vi "FPGAcode4_NoInit.vi"() -> ()   [LabVIEW 2015]
uses:
  Limits_In.ctl
  Detector_Cluster.ctl
  <vilib>/Platform/TimedLoop/XDataNode/timing_clust.ctl
  <vilib>/Platform/TimedLoop/XDataNode/nitl_modes.ctl
  <vilib>/Platform/TimedLoop/XDataNode/wakeup.ctl
  Correlations.ctl
  <vilib>/rvi/Emulation/niFpgaSctlEmulationGetInTimedLoop.vi
  <vilib>/rvi/Emulation/niFpgaEmulationReportErrorSimple.vi
  <vilib>/rvi/Emulation/niFpgaGetClockAttributes.vi
  <vilib>/rvi/Emulation/niFpgaCriticalErrorInLSC.vi
  <vilib>/rvi/eio/common/nirviEmuTemplateMethod_errors.vi
  <vilib>/rvi/Emulation/niFpgaEmulationIsFPGAContextNoSignature.vi
  <vilib>/rvi/DataTransferAndStorage/Container/Common/niFpgaContainerGetUniqueNameForEmu.vi
  <vilib>/rvi/eio/common/nirviEmuReportErrorAndStop.vi
  <vilib>/rvi/Emulation/niFpgaProcessEmulError.vi
  <vilib>/Platform/TimedLoop/XDataNode/XDataNode.xnode
  <vilib>/eio/EIONode/EIONode.xnode
  <vilib>/rvi/DataTransferAndStorage/Container/XNode/niFpgaContainer.xnode
  <vilib>/rvi/DataTransferAndStorage/Handshake/Emulation/niFpgaHandshakeEmulation.vi
  <vilib>/Platform/TimedLoop/XDataNode/XDNodeRunTimeDep.lvlib
panel:
  in  "User Trigger?":bool
  in  "User Trigger Distance":fxp<+/-,34,18> format="%.3g"
  in  "Charge Error Factor":fxp<+,32,0>=0.19999999995343387 format="%_2g"
  in  "Threshold Factor":fxp<+/-,32,16>=1.149993896484375 format="%.2g"
  in  "Limits":T1={"High Charge Limit"=4.54747350780585e-13, "Low Charge Limit"=0.0, "High Velocity Limit"=262143.0, "Low Velocity Limit"=0.0, "High Mass Limit"=7.27595761248936e-12, "Low Mass Limit"=0.0, "High Voltage"=2200000.0}
  in  "Calibrate":bool=TRUE
  in  "Armed":bool
  in  "One Shot":bool
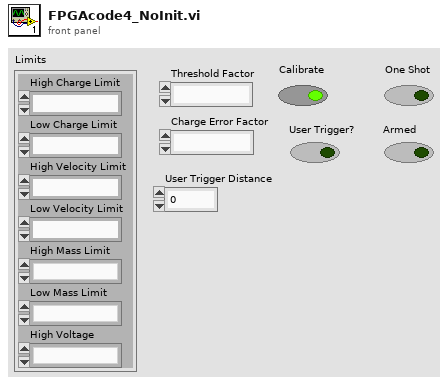
[diagram p1: front panel]
types:
  T1 = typedef "Limits_In.ctl" = cluster{"High Charge Limit":fxp<+,32,-41>, "Low Charge Limit":fxp<+,32,-41>, "High Velocity Limit":fxp<+,18,18>, "Low Velocity Limit":fxp<+,18,18>, "High Mass Limit":fxp<+,32,-37>, "Low Mass Limit":fxp<+,32,-37>, "High Voltage":fxp<+,32,22>}
  T2 = cluster{"[0]":fxp<+,16,1>, "[1]":fxp<+,16,1>, "[2]":fxp<+,16,1>, "[3]":fxp<+,16,1>, "[4]":fxp<+,16,1>, "[5]":fxp<+,16,1>, "[6]":fxp<+,16,1>, "[7]":fxp<+,16,1>, "[8]":fxp<+,16,1>, "[9]":fxp<+,16,1>, "[10]":fxp<+,16,1>}
  T3 = cluster{"[0]":i32, "[1]":i32, "[2]":i32, "[3]":i32, "[4]":i32, "[5]":i32, "[6]":i32, "[7]":i32, "[8]":i32, "[9]":i32, "[10]":i32}
  T4 = cluster{"[0]":cluster{"Detector Max Speed Count":i32, "Detector Min Speed Count":i32, "Gap Max Speed Count":i32, "Gap Min Speed Count":i32}, "[1]":cluster{"Detector Max Speed Count":i32, "Detector Min Speed Count":i32, "Gap Max Speed Count":i32, "Gap Min Speed Count":i32}, "[2]":cluster{"Detector Max Speed Count":i32, "Detector Min Speed Count":i32, "Gap Max Speed Count":i32, "Gap Min Speed Count":i32}, "[3]":cluster{"Detector Max Speed Count":i32, "Detector Min Speed Count":i32, "Gap Max Speed Count":i32, "Gap Min Speed Count":i32}, "[4]":cluster{"Detector Max Speed Count":i32, "Detector Min Speed Count":i32, "Gap Max Speed Count":i32, "Gap Min Speed Count":i32}, "[5]":cluster{"Detector Max Speed Count":i32, "Detector Min Speed Count":i32, "Gap Max Speed Count":i32, "Gap Min Speed Count":i32}, "[6]":cluster{"Detector Max Speed Count":i32, "Detector Min Speed Count":i32, "Gap Max Speed Count":i32, "Gap Min Speed Count":i32}, "[7]":cluster{"Detector Max Speed Count":i32, "Detector Min Speed Count":i32, "Gap Max Speed Count":i32, "Gap Min Speed Count":i32}, "[8]":cluster{"Detector Max Speed Count":i32, "Detector Min Speed Count":i32, "Gap Max Speed Count":i32, "Gap Min Speed Count":i32}, "[9]":cluster{"Detector Max Speed Count":i32, "Detector Min Speed Count":i32, "Gap Max Speed Count":i32, "Gap Min Speed Count":i32}, "[10]":cluster{"Detector Max Speed Count":i32, "Detector Min Speed Count":i32, "Gap Max Speed Count":i32, "Gap Min Speed Count":i32}}
  T5 = cluster{cluster{"[0]":i32, "[1]":i32, "[2]":i32, "[3]":i32, "[4]":i32, "[5]":i32, "[6]":i32, "[7]":i32, "[8]":i32, "[9]":i32, "[10]":i32}, cluster{"[0]":i32, "[1]":i32, "[2]":i32, "[3]":i32, "[4]":i32, "[5]":i32, "[6]":i32, "[7]":i32, "[8]":i32, "[9]":i32, "[10]":i32}, cluster{"[0]":i32, "[1]":i32, "[2]":i32, "[3]":i32, "[4]":i32, "[5]":i32, "[6]":i32, "[7]":i32, "[8]":i32, "[9]":i32, "[10]":i32}, cluster{"[0]":i32, "[1]":i32, "[2]":i32, "[3]":i32, "[4]":i32, "[5]":i32, "[6]":i32, "[7]":i32, "[8]":i32, "[9]":i32, "[10]":i32}}
  T6 = cluster{"Distance to PSU":fxp<+/-,64,37>, "Distance to end of PSU":fxp<+/-,64,37>, "Distance to DCS 2":fxp<+/-,64,37>, "Distance to DCS 1":fxp<+/-,64,37>, "Distance to front of LEIL Chamber":fxp<+/-,64,37>}
  T7 = typedef "Detector_Cluster.ctl" = cluster{"Det 1":i32, "Det 2":i32}
  T8 = cluster{"Filter 1":T7, "Filter 2":T7, "Filter 3":T7, "Filter 4":T7}
  T9 = cluster{"Detector Max Speed Count":i32, "Detector Min Speed Count":i32, "Gap Max Speed Count":i32, "Gap Min Speed Count":i32}[]
  T10 = cluster{"Filter 1":T7, "Filter 2":T7, "Filter 3":T7, "Filter 4":T7}[]
  T11 = typedef "XDNodeRunTimeDep.lvlib/timing_clust.ctl" = cluster{"Expected End [f-1]":u64, "Actual End [f-1]":u64, "Finished Late? [f-1]":bool, "Expected End [i-1]":u64, "Actual End [i-1]":u64, "Finished Late? [i-1]":bool, "Expected Start [i]":u64, "Actual Start [i]":u64, "Expected Start [f]":u64, "Actual Start [f]":u64, "Source Name":string, "Structure Name":string, "Period":i64, "Deadline":i64, "Offset":i64, "Start":i64, "Priority":i32, "Timeout":i32, "Mode":T12, "Wakeup Reason":T13, "Error":errorcluster, "Source Type":string, "Secondary Source Type":string, "Global End Time":u64, "Global Start Time":u64, "Frame Duration":u64, "Iteration Duration":u64, "Assigned CPU":i32, "I/O Scan Engine Mode":u32}
  T12 = typedef "XDNodeRunTimeDep.lvlib/nitl_modes.ctl" = enum32{"No Change", "Process missed periods, maintain original phase", "Discard missed periods, maintain original phase", "Process missed periods, ignore original phase", "Discard missed periods, ignore original phase"}
  T13 = typedef "XDNodeRunTimeDep.lvlib/wakeup.ctl" = enum32{"Normal", "Aborted", "Asynchronous wakeup", "Timing source error", "Timed loop error", "Timeout"}
  T14 = cluster{"First Detector Count":i32, "Detector Gap Count":i32, "Second Detector Count":i32, "Second Detector Final Count":i32}
  T15 = typedef "Correlations.ctl" = cluster{"First Correlation":i32, "Latest Correlation":i32}
  T16 = cluster{"Data":fxp<+/-,35,32>, "Data":fxp<+/-,35,32>}
  T17 = cluster{cluster{"Data":i16, "Data":i16}, cluster{"Det 1":i16, "Det 2":i16}, cluster{"Det 1":i16, "Det 2":i16}, cluster{"Det 1":i16, "Det 2":i16}}
  T18 = cluster{cluster{"Det 1":i16, "Det 2":i16}, cluster{"Det 1":i16, "Det 2":i16}, cluster{"Det 1":i16, "Det 2":i16}, cluster{"Det 1":i16, "Det 2":i16}}
  T19 = cluster{"Distance to PSU":fxp<+/-,64,69>, "Distance to end of PSU":fxp<+/-,64,69>, "Distance to DCS 2":fxp<+/-,64,69>, "Distance to DCS 1":fxp<+/-,64,69>, "Distance to front of LEIL Chamber":fxp<+/-,64,69>}
  T20 = cluster{"Distance to PSU":i32, "Distance to end of PSU":i32, "Distance to DCS 2":i32, "Distance to DCS 1":i32, "Distance to front of LEIL Chamber":i32}
  T21 = cluster{"IO Module\\AI 0":i16, "IO Module\\AI 1":i16}
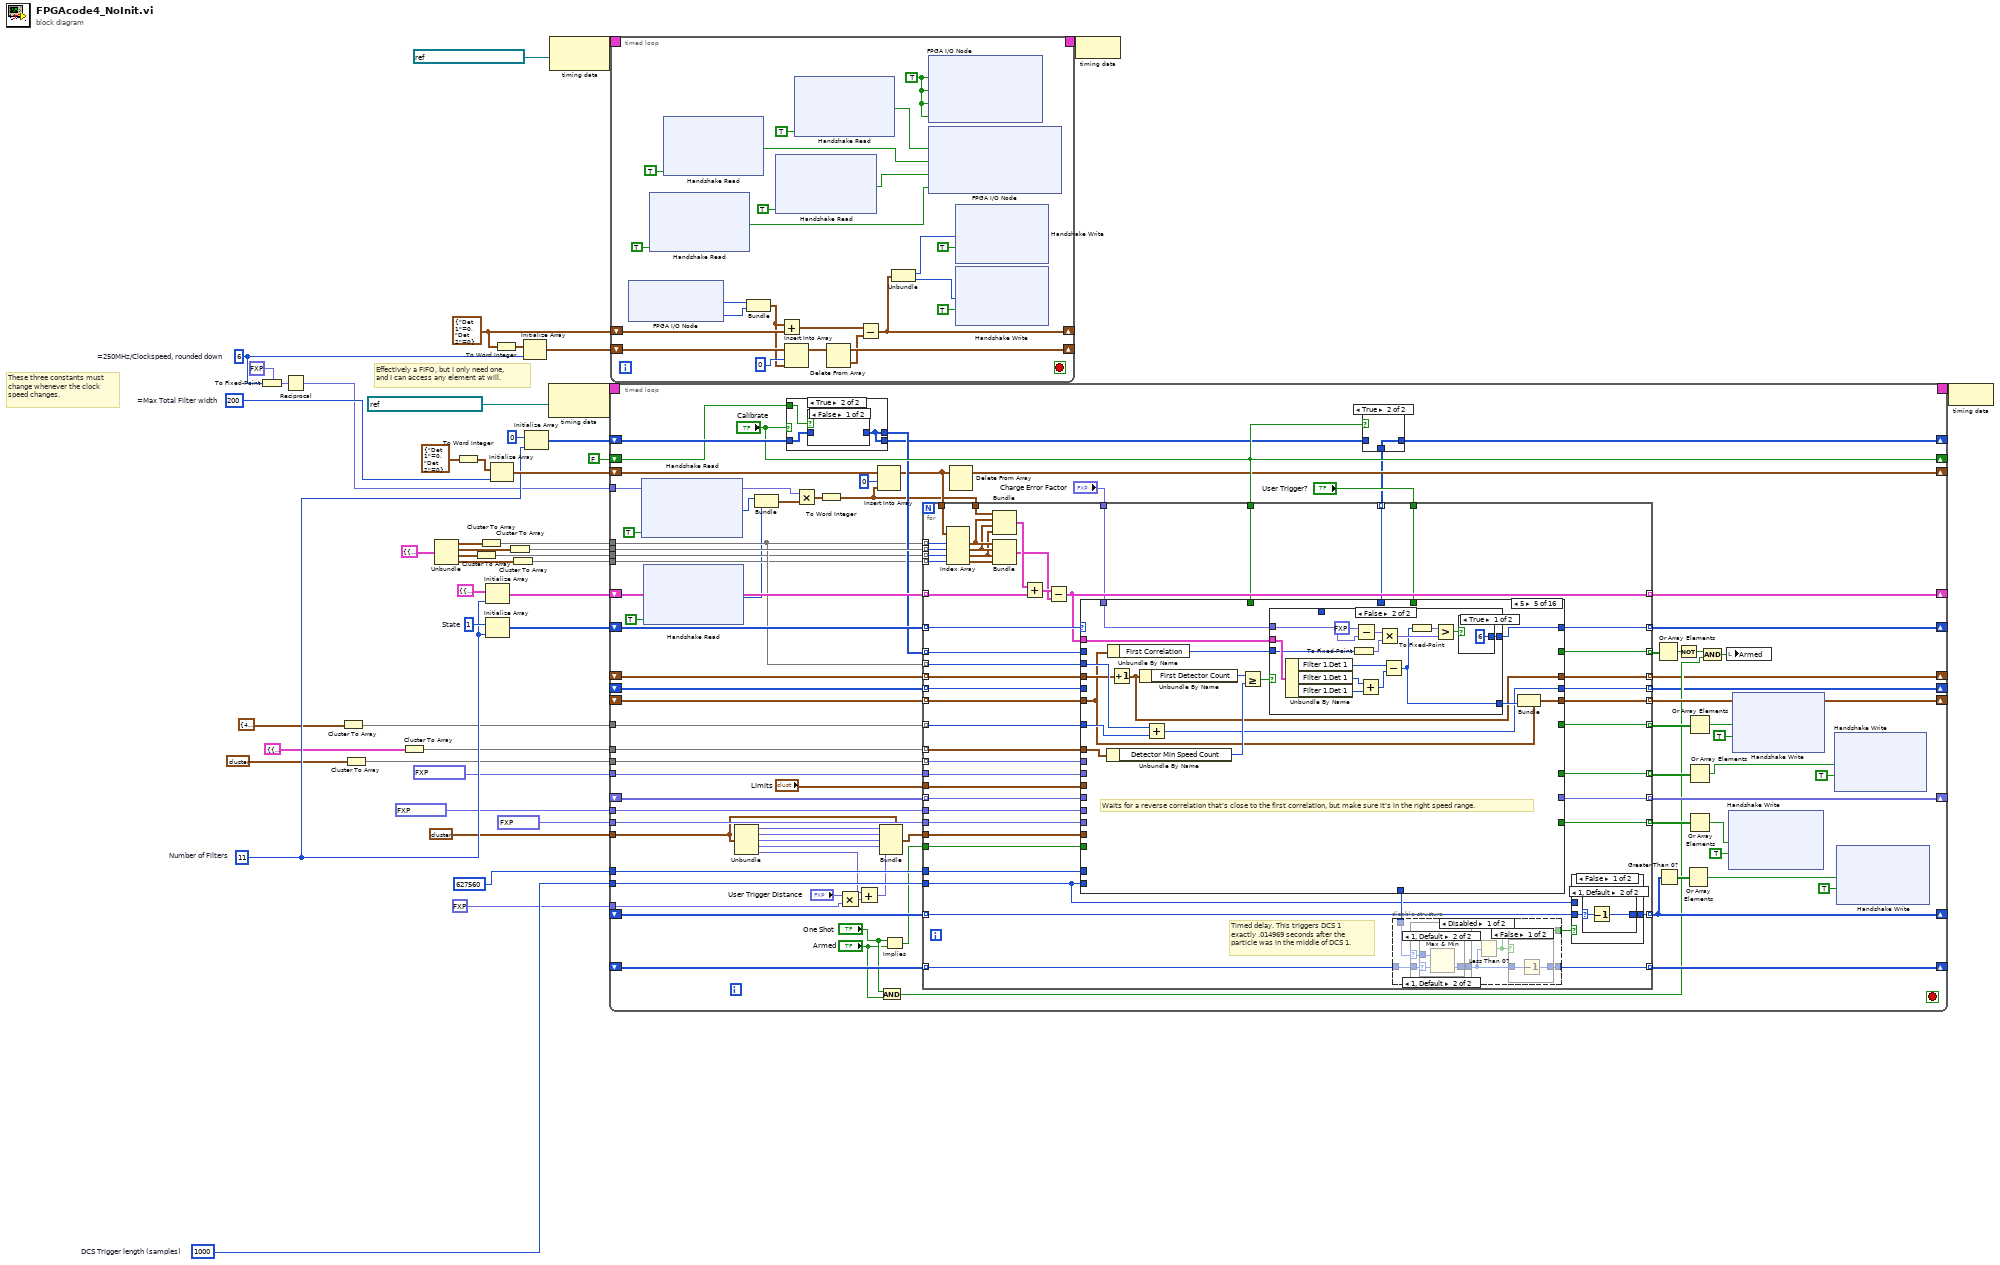
[diagram p0: block diagram]
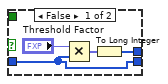
[diagram p2: hidden frame]
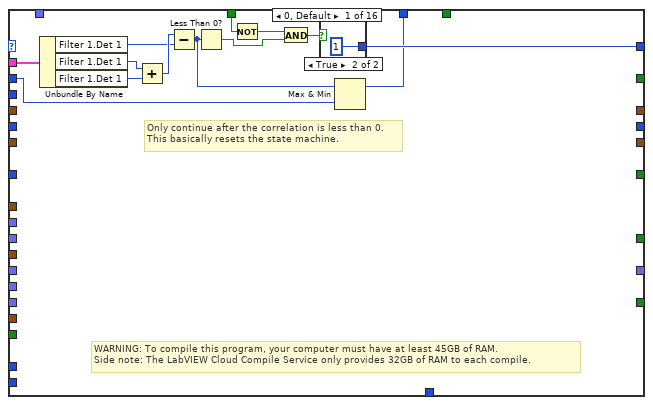
[diagram p5: hidden frame]
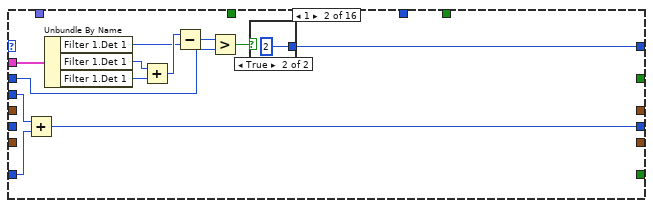
[diagram p7: hidden frame]
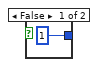
[diagram p8: hidden frame]
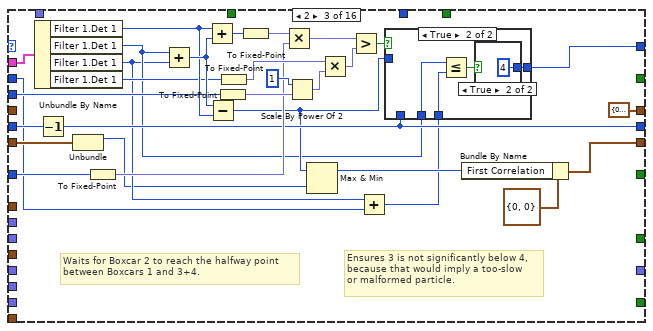
[diagram p9: hidden frame]
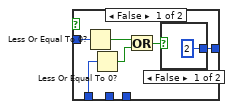
[diagram p10: hidden frame]
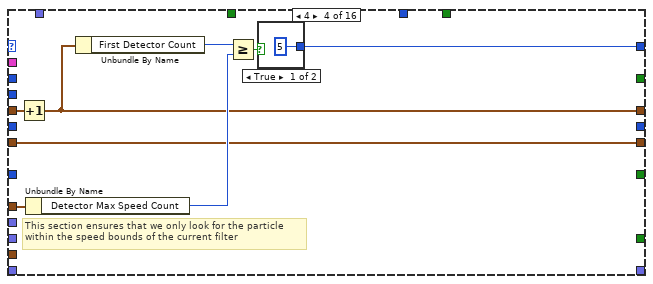
[diagram p13: hidden frame]
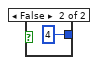
[diagram p14: hidden frame]
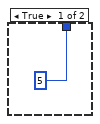
[diagram p15: hidden frame]
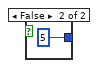
[diagram p16: hidden frame]
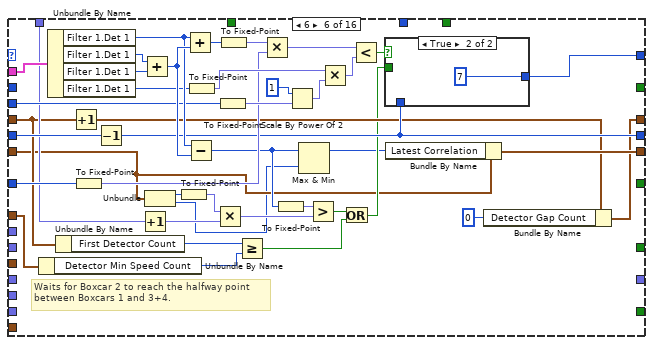
[diagram p17: hidden frame]
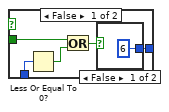
[diagram p18: hidden frame]
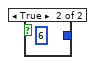
[diagram p19: hidden frame]
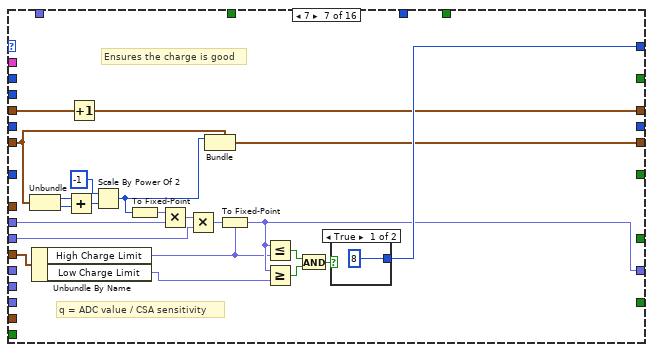
[diagram p20: hidden frame]
diagram:
  w27 = T7 {"Det 1"=0, "Det 2"=0} ("Detectors")
  w24 = u8 6  # =250MHz/Clockspeed, rounded down
  w33 = 200  # =Max Total Filter width
  w40 = u16 1000  # DCS Trigger length (samples)
  w46 = u8 1  # State
  w34 = 11  # Number of Filters
  # "These three constants must\nchange whenever the clock\nspeed changes."
  # "Effectively a FIFO, but I only need one,\nand I can access any element at will."
  n1 = To Fixed-Point(fixed-point type=fxp<+,3,3> 0.0, number=w24) -> (fixed-point=w30:fxp<+,3,3>)
  n2 = Reciprocal(x=w30) -> (1/x=w28:fxp<+,4,1>)
  n3 = Cluster To Array(cluster=T3 {"[0]"=4000, "[1]"=2359, "[2]"=1391, "[3]"=820, "[4]"=484, "[5]"=285, "[6]"=168, "[7]"=99, "[8]"=59, "[9]"=35, "[10]"=20}) -> (array=w7:i32[])
  n4 = Cluster To Array(cluster=T2 {"[0]"=0.000823974609375, "[1]"=0.000823974609375, "[2]"=0.000823974609375, "[3]"=0.000823974609375, "[4]"=0.000823974609375, "[5]"=0.00152587890625, "[6]"=0.003265380859375, "[7]"=0.007080078125, "[8]"=0.015869140625, "[9]"=0.03704833984375, "[10]"=0.100006103515625} ("cluster 3")) -> (array=w5:fxp<+,16,1>[])
  n5 = Cluster To Array(cluster=T4 {"[0]"={"Detector Max Speed Count"=42000, "Detector Min Speed Count"=84000, "Gap Max Speed Count"=78000, "Gap Min Speed Count"=156000}, "[1]"={"Detector Max Speed Count"=21477, "Detector Min Speed Count"=42953, "Gap Max Speed Count"=39885, "Gap Min Speed Count"=79770}, "[2]"={"Detector Max Speed Count"=10982, "Detector Min Speed Count"=21964, "Gap Max Speed Count"=20395, "Gap Min Speed Count"=40790}, "[3]"={"Detector Max Speed Count"=5616, "Detector Min Speed Count"=11231, "Gap Max Speed Count"=10429, "Gap Min Speed Count"=20858}, "[4]"={"Detector Max Speed Count"=2872, "Detector Min Speed Count"=5743, "Gap Max Speed Count"=5333, "Gap Min Speed Count"=10666}, "[5]"={"Detector Max Speed Count"=1468, "Detector Min Speed Count"=2937, "Gap Max Speed Count"=2727, "Gap Min Speed Count"=5454}, "[6]"={"Detector Max Speed Count"=751, "Detector Min Speed Count"=1502, "Gap Max Speed Count"=1394, "Gap Min Speed Count"=2789}, "[7]"={"Detector Max Speed Count"=384, "Detector Min Speed Count"=768, "Gap Max Speed Count"=713, "Gap Min Speed Count"=1426}, "[8]"={"Detector Max Speed Count"=196, "Detector Min Speed Count"=393, "Gap Max Speed Count"=365, "Gap Min Speed Count"=729}, "[9]"={"Detector Max Speed Count"=100, "Detector Min Speed Count"=201, "Gap Max Speed Count"=186, "Gap Min Speed Count"=373}, "[10]"={"Detector Max Speed Count"=51, "Detector Min Speed Count"=103, "Gap Max Speed Count"=95, "Gap Min Speed Count"=191}} ("cluster 2")) -> (array=w4:T9)
  n6 = Unbundle(T5 {{"[0]"=1200, "[1]"=1200, "[2]"=1200, "[3]"=1200, "[4]"=1200, "[5]"=650, "[6]"=306, "[7]"=140, "[8]"=62, "[9]"=26, "[10]"=10}, {"[0]"=5200, "[1]"=3559, "[2]"=2591, "[3]"=2020, "[4]"=1684, "[5]"=935, "[6]"=474, "[7]"=240, "[8]"=122, "[9]"=62, "[10]"=30}, {"[0]"=5800, "[1]"=4159, "[2]"=3191, "[3]"=2620, "[4]"=2284, "[5]"=1260, "[6]"=627, "[7]"=310, "[8]"=153, "[9]"=75, "[10]"=35}, {"[0]"=6400, "[1]"=4759, "[2]"=3791, "[3]"=3220, "[4]"=2884, "[5]"=1585, "[6]"=780, "[7]"=380, "[8]"=184, "[9]"=88, "[10]"=40}} ("output cluster")) -> (w21:T3, w20:T3, w19:T3, w18:T3)
  n7 = To Word Integer(number=T7 {"Det 1"=0, "Det 2"=0} ("Detectors")) -> (16bit integer=w43:cluster{"Det 1":i16, "Det 2":i16})
  n8 = Cluster To Array(cluster=w19) -> (array=w9:i32[])
  n9 = Cluster To Array(cluster=w21) -> (array=w11:i32[])
  n10 = Initialize Array(T8 {"Filter 1"={"Det 1"=0, "Det 2"=0}, "Filter 2"={"Det 1"=0, "Det 2"=0}, "Filter 3"={"Det 1"=0, "Det 2"=0}, "Filter 4"={"Det 1"=0, "Det 2"=0}} ("cluster"), w34) -> (w44:T10)
  n11 = Initialize Array(w46, w34) -> (w45:u8[])
  n12 = Initialize Array(w43, w33) -> (w47:cluster{"Det 1":i16, "Det 2":i16}[])
  n13 = To Word Integer(number=w27) -> (16bit integer=w26:cluster{"Det 1":i16, "Det 2":i16})
  n14 = Cluster To Array(cluster=w20) -> (array=w10:i32[])
  n15 = Cluster To Array(cluster=w18) -> (array=w8:i32[])
  n16 = Initialize Array(w26, w24) -> (w25:cluster{"Det 1":i16, "Det 2":i16}[])
  n17 = Initialize Array(0 ("Thresholds in"), w34) -> (w35:i32[])
  n18 = node-c288(refnum<k21> "40 MHz Onboard Clock" ("Source Name")) -> (w39:T11)
  n19 = node-c288(refnum<k21> "IO Module\\Data Clock" ("Source Name")) -> (w32:T11)
  n20 = timed-loop {
    shift-right: [w65] -> _
    shift-left: w47 -> [w128]
    shift-right: [w73] -> _
    shift-left: w44 -> [w125]
    shift-right: [w67] -> _
    shift-left: w45 -> [w127]
    shift-right: [w74] -> _
    shift-left: _ -> [w126]
    tunnel: w4 -> [w124]
    shift-right: [w123] -> _
    shift-left: _ -> [w122]
    tunnel: w11 -> [w72]
    tunnel: w10 -> [w121]
    tunnel: w7 -> [w120]
    tunnel: w5 -> [w119]
    shift-right: [w118] -> _
    shift-left: _ -> [w117]
    tunnel: fxp<+,32,-43> 9.525990075777386e-16 ("fixed-point 2") -> [w116]
    tunnel: fxp<+,32,-49> 2.2727300016438096e-16 ("fixed-point 3") -> [w115]
    tunnel: fxp<+,28,28> 32400000.0 ("fixed-point") -> [w114]
    tunnel: T6 {"Distance to PSU"=1.2345678955316544, "Distance to end of PSU"=2.4691357985138893, "Distance to DCS 2"=3.229876533150673, "Distance to DCS 1"=-1.677654318511486, "Distance to front of LEIL Chamber"=5.305777758359909} ("x/y") -> [w103]
    shift-right: [w113] -> _
    shift-left: w35 -> [w112]
    shift-right: ["Calibrate"] -> _
    shift-left: FALSE ("Calibrate") -> [w111]
    tunnel: w40 -> [w110]
    tunnel: 627560 ("32bit integer") -> [w109]
    shift-right: [w107] -> _
    shift-left: _ -> [w108]
    shift-right: [w106] -> _
    shift-left: _ -> [w105]
    tunnel: fxp<+/-,34,33> 1.0 ("1/x") -> [w104]
    shift-right: [w71] -> _
    shift-left: _ -> [w70]
    tunnel: w8 -> [w69]
    tunnel: w9 -> [w68]
    timing: w39 -> [_]
    timing-out: [_] -> w38
    tunnel: w28 -> [w63]
    stop <- _ stop-if-true
    n21 = xnode ("Handshake Read")("Ready for Output"=TRUE) -> ("Data"=w50:i32)  [unwired: 1 in, 2 out]
    n22 = xnode ("Handshake Read")("Ready for Output"=TRUE) -> ("Data"=w49:i32)  [unwired: 1 in, 2 out]
    n23 = Unbundle(w103) -> ("Distance to PSU"=w96:fxp<+/-,64,37>, "Distance to end of PSU"=w95:fxp<+/-,64,37>, "Distance to DCS 2"=w94:fxp<+/-,64,37>, "Distance to DCS 1"=w91:fxp<+/-,64,37>, "Distance to front of LEIL Chamber"=w90:fxp<+/-,64,37>)
    n24 = Bundle("Data"=w50, "Data"=w49) -> (w48:cluster{"Data":i32, "Data":i32})  [unwired: 1 in]
    n25 = case shown="True" "Calibrate" {
      tunnel: w112 -> [w130 w134]
      tunnel: [w130 w133] -> w75
      tunnel: w111 -> [_ w135]
      tunnel: [w129 w133] -> w76
      frame False {
        n26 = Multiply(x="Threshold Factor", y=w130) -> (x*y=w131:fxp<+/-,64,48>[])
        n27 = To Long Integer(number=w131) -> (32bit integer=w129:i32[])
      }
      frame True {
        n28 = case shown="False" w135 {
          tunnel: w134 -> [_ w136]
          tunnel: [_ w136] -> w133
          frame False {
          }
          frame True {
          }
        }
      }
    }
    n29 = Multiply(x=w63, y=w48) -> (x*y=w64:T16)
    n30 = To Word Integer(number=w64) -> (16bit integer=w62:cluster{"Data":i16, "Data":i16})
    n31 = Multiply(x="User Trigger Distance", y=w104) -> (x*y=w92:fxp<+/-,64,49>)
    n32 = Add(x=w90, y=w92) -> (x+y=w89:fxp<+/-,64,50>)
    n33 = Insert Into Array(array=w128, index=0, new element=w62) -> (w66:cluster{"Det 1":i16, "Det 2":i16}[])
    n34 = Bundle(cluster=w103, "Distance to PSU"=w96, "Distance to end of PSU"=w95, "Distance to DCS 2"=w94, "Distance to DCS 1"=w91, "Distance to front of LEIL Chamber"=w89) -> (w93:T6)
    n35 = And(x="One Shot", y="Armed") -> (x .and. y?=w82:bool)
    n36 = Implies(1:"Armed", 2:"One Shot") -> (0:w99:bool)
    n37 = for {
      tunnel: w66 -> [w190]
      tunnel: [w176] -> w73 mode=indexing
      tunnel: w127 -> [w189] mode=indexing
      tunnel: [w188] -> w67 mode=indexing
      tunnel: w76 -> [w143] mode=indexing
      tunnel: [w187] -> w74 mode=indexing
      tunnel: w126 -> [w186] mode=indexing
      tunnel: w125 -> [w180] mode=indexing
      tunnel: w62 -> [w185]
      tunnel: w124 -> [w175] mode=indexing
      tunnel: [w174] -> w123 mode=indexing
      tunnel: w122 -> [w173] mode=indexing
      tunnel: w72 -> [w172] mode=indexing
      tunnel: w121 -> [w141] mode=indexing
      tunnel: w68 -> [w171] mode=indexing
      tunnel: w69 -> [w170] mode=indexing
      tunnel: w72 -> [w145] mode=indexing
      tunnel: w120 -> [w144] mode=indexing
      tunnel: "Charge Error Factor" -> [w169]
      tunnel: w119 -> [w168] mode=indexing
      tunnel: "Limits" -> [w167]
      tunnel: [w166] -> w118 mode=indexing
      tunnel: w117 -> [w165] mode=indexing
      tunnel: w116 -> [w164]
      tunnel: w115 -> [w163]
      tunnel: w114 -> [w162]
      tunnel: w93 -> [w161]
      tunnel: w99 -> [w160]
      tunnel: w110 -> [w157]
      tunnel: w109 -> [w159]
      tunnel: [w156] -> w107 mode=indexing
      tunnel: w108 -> [w155] mode=indexing
      tunnel: [w153] -> w106 mode=indexing
      tunnel: w105 -> [w152] mode=indexing
      tunnel: [w151] -> w88 mode=indexing
      tunnel: [w150] -> w87 mode=indexing
      tunnel: [w149] -> w86 mode=indexing
      tunnel: [w148] -> w85 mode=indexing
      tunnel: "User Trigger?" -> [w147]
      tunnel: "Calibrate" -> [w146]
      tunnel: [w142] -> w71 mode=indexing
      tunnel: w70 -> [w140] mode=indexing
      tunnel: [w139] -> w61 mode=indexing
      # "Timed delay. This triggers DCS 1\nexactly .014969 seconds after the\nparticle was in the middle of DCS 1."
      n38 = Index Array(array=w190, index #1=w172, index #2=w141, index #3=w171, index #4=w170) -> (element #1=w183:cluster{"Det 1":i16, "Det 2":i16}, element #2=w182:cluster{"Det 1":i16, "Det 2":i16}, element #3=w181:cluster{"Det 1":i16, "Det 2":i16}, element #4=w184:cluster{"Det 1":i16, "Det 2":i16})
      n39 = Bundle(w185, w183, w182, w181) -> (w179:T17)  [unwired: 1 in]
      n40 = Bundle(w183, w182, w181, w184) -> (w177:T18)  [unwired: 1 in]
      n41 = Add(x=w179, y=w180) -> (x+y=w178:T8)
      n42 = Subtract(x=w178, y=w177) -> (x-y=w176:T8)
      n43 = case shown="5" w189 {
        tunnel: w143 -> [w193 w216 w222 _ _ _ _ _ _ _ _ _ _ _ _ _]
        tunnel: [w202 w215 w247 w264 w279 w345 w367 w381 w395 w458 w471 w485 w546 w573 u8 16 ("Det 3") w632] -> w188
        tunnel: w145 -> [_ w208 w241 _ w281 w337 _ _ w397 w450 _ w487 w538 _ w606 _]
        tunnel: [_ _ T14 {"First Detector Count"=0, "Detector Gap Count"=0, "Second Detector Count"=0, "Second Detector Final Count"=0} ("Cutoffs") w261 w271 w308 w357 w378 w389 w422 w468 w480 w526 w556 w595 w630] -> w187
        tunnel: w186 -> [_ _ _ w262 w276 w313 w358 w379 w392 w428 w469 w482 w516 w556 w594 w631]
        tunnel: w140 -> [_ _ w248 _ _ w346 _ _ _ w459 _ _ w547 _ _ _]
        tunnel: w176 -> [w197 w210 w234 _ w282 w330 _ _ w398 w444 _ w488 w532 _ _ _]
        tunnel: w175 -> [_ _ _ w268 w286 w314 _ w385 w402 w427 w475 w492 w517 _ _ _]
        tunnel: w173 -> [_ _ w225 w263 w273 w312 w360 w380 w391 w437 w470 w478 w510 _ _ _]
        tunnel: w144 -> [_ w207 w242 _ w280 w338 _ _ w396 w451 _ w486 w539 _ w598 _]
        tunnel: w169 -> [_ _ _ _ w283 w323 _ _ w399 w438 _ w489 w525 _ _ _]
        tunnel: w168 -> [_ _ _ _ _ _ w372 _ _ _ _ _ _ _ _ _]
        tunnel: w167 -> [_ _ _ _ _ _ w375 _ _ _ _ _ _ w584 _ _]
        tunnel: [_ _ _ _ _ _ w355 w377 w388 w420 w467 w479 w511 _ _ _] -> w166
        tunnel: w165 -> [_ _ _ _ _ _ _ w377 w388 w420 w467 w479 w511 w562 _ _]
        tunnel: w164 -> [_ _ _ _ _ _ _ _ _ _ _ _ _ w583 _ _]
        tunnel: w163 -> [_ _ _ _ _ _ w365 _ _ _ _ _ _ _ _ _]
        tunnel: w162 -> [_ _ _ _ _ _ _ _ _ _ _ _ _ w561 _ _]
        tunnel: w161 -> [_ _ _ _ _ _ _ _ _ _ _ _ _ _ w609 _]
        tunnel: w160 -> [_ _ _ _ _ _ _ _ _ _ _ _ _ w567 _ _]
        tunnel: w159 -> [_ _ _ _ _ _ _ _ _ _ _ _ _ _ w603 _]
        tunnel: w157 -> [_ _ _ _ _ _ _ _ _ _ _ _ _ _ _ w629]
        tunnel: [_ _ _ _ _ _ _ _ _ _ _ _ _ _ w601 _] -> w158
        tunnel: [_ _ _ _ _ _ _ _ _ _ _ _ _ _ _ w628] -> w151
        tunnel: [_ _ _ _ _ _ _ _ _ _ _ _ _ _ _ w627] -> w150
        tunnel: [_ _ _ _ _ _ _ _ _ _ _ _ _ _ _ w626] -> w149
        tunnel: [_ _ _ _ _ _ _ _ _ _ _ _ _ w566 _ _] -> w148
        tunnel: w147 -> [_ _ _ _ _ _ _ _ _ _ _ _ _ _ _ w611]
        tunnel: w146 -> [w195 _ _ _ _ _ _ _ _ _ _ _ _ _ _ _]
        tunnel: [_ w206 w230 _ w272 w326 _ _ w390 w440 _ w481 w528 _ _ _] -> w142
        tunnel: [_ _ w236 w263 w275 w332 w359 w380 w391 w437 w470 w478 w510 _ _ _] -> w174
        tunnel: [w191 _ _ _ _ _ _ _ _ _ _ _ _ _ _ _] -> w139
        frame 0, Default {
          # "WARNING: To compile this program, your computer must have at least 45GB of RAM.\nSide note: The LabVIEW Cloud Compile Service only provides 32GB of RAM to each compile."
          # "Only continue after the correlation is less than 0.\nThis basically resets the state machine."
          n44 = Unbundle By Name(w197) -> ("Filter 1.Det 1"=w198:i32, "Filter 1.Det 1"=w199:i32, "Filter 1.Det 1"=w200:i32)
          n45 = Add(x=w199, y=w200) -> (x+y=w201:i32)
          n46 = Subtract(x=w201, y=w198) -> (x-y=w192:i32)
          n47 = Less Than 0?(x=w192) -> (x < 0?=w203:bool)
          n48 = Not(x=w195) -> (.not. x?=w194:bool)
          n49 = And(x=w194, y=w203) -> (x .and. y?=w196:bool)
          n50 = case shown="True" w196 {
            tunnel: [_ u8 1 ("Det 3")] -> w202
            frame False {
            }
            frame True {
            }
          }
          n51 = Max & Min(x=w192, y=w193) -> (max(x,y)=w191:i32)  [unwired: 1 out]
        }
        frame 1 {
          n52 = Add(x=w208, y=w207) -> (x+y=w206:i32)
          n53 = Unbundle By Name(w210) -> ("Filter 1.Det 1"=w211:i32, "Filter 1.Det 1"=w212:i32, "Filter 1.Det 1"=w213:i32)
          n54 = Add(x=w212, y=w213) -> (x+y=w214:i32)
          n55 = Subtract(x=w214, y=w211) -> (x-y=w209:i32)
          n56 = Greater?(x=w209, y=w216) -> (0:w205:bool)
          n57 = case shown="True" w205 {
            tunnel: [u8 1 ("Det 3") u8 2 ("Det 3")] -> w215
            frame False {
            }
            frame True {
            }
          }
        }
        frame 2 {
          # "Ensures 3 is not significantly below 4,\nbecause that would imply a too-slow\nor malformed particle."
          # "Waits for Boxcar 2 to reach the halfway point\nbetween Boxcars 1 and 3+4."
          n58 = Unbundle By Name(w234) -> ("Filter 1.Det 1"=w244:i32, "Filter 1.Det 1"=w221:i32, "Filter 1.Det 1"=w220:i32, "Filter 1.Det 1"=w238:i32)
          n59 = Decrement(x=w248) -> (x-1=w230:i32)
          n60 = Unbundle(w225) -> ("First Correlation"=w219:i32)  [unwired: 1 out]
          n61 = To Fixed-Point(number=w242) -> (fixed-point=w231:fxp<+/-,32,32>)  [unwired: 1 in]
          n62 = Add(x=w221, y=w220) -> (x+y=w245:i32)
          n63 = Add(x=w244, y=w245) -> (x+y=w246:i32)
          n64 = Subtract(x=w245, y=w244) -> (x-y=w226:i32)
          n65 = To Fixed-Point(number=w241) -> (fixed-point=w232:fxp<+/-,32,32>)  [unwired: 1 in]
          n66 = To Fixed-Point(number=w238) -> (fixed-point=w233:fxp<+/-,32,32>)  [unwired: 1 in]
          n67 = To Fixed-Point(number=w246) -> (fixed-point=w235:fxp<+/-,32,32>)  [unwired: 1 in]
          n68 = Multiply(x=w235, y=w231) -> (x*y=w243:fxp<+/-,64,64>)
          n69 = Scale By Power Of 2(n=i16 1, x=w232) -> (x*2^n=w239:fxp<+/-,32,32>)
          n70 = Max & Min(x=w226, y=w219) -> (max(x,y)=w227:i32)  [unwired: 1 out]
          n71 = Multiply(x=w233, y=w239) -> (x*y=w237:fxp<+/-,64,64>)
          n72 = Greater?(x=w243, y=w237) -> (0:w228:bool)
          n73 = Add(x=w220, y=w222) -> (x+y=w223:i32)
          n74 = case shown="True" w228 {
            tunnel: [w254 w259] -> w247
            tunnel: w230 -> [w250 _]
            tunnel: w226 -> [w249 _]
            tunnel: w223 -> [_ w257]
            tunnel: w221 -> [_ w258]
            frame False {
              n75 = Less Or Equal To 0?(x=w249) -> (x <= 0?=w252:bool)
              n76 = Less Or Equal To 0?(x=w250) -> (x <= 0?=w251:bool)
              n77 = Or(x=w252, y=w251) -> (x .or. y?=w253:bool)
              n78 = case shown="False" w253 {
                tunnel: [u8 2 ("Det 3") _] -> w254
                frame False {
                }
                frame True {
                }
              }
            }
            frame True {
              n79 = Less Or Equal?(x=w258, y=w257) -> (x <= y?=w256:bool)
              n80 = case shown="True" w256 {
                tunnel: [_ u8 4 ("Det 3")] -> w259
                frame False {
                }
                frame True {
                }
              }
            }
          }
          n81 = Bundle By Name(cluster=T15 {"First Correlation"=0, "Latest Correlation"=0}, "First Correlation"=w227) -> (w236:T15)
        }
        frame 4 {
          # "This section ensures that we only look for the particle\nwithin the speed bounds of the current filter"
          n82 = Increment(x=w262) -> (x+1=w261:T14)
          n83 = Unbundle By Name(w268) -> ("Detector Max Speed Count"=w266:i32)
          n84 = Unbundle By Name(w261) -> ("First Detector Count"=w267:i32)
          n85 = Greater Or Equal?(x=w267, y=w266) -> (x >= y?=w265:bool)
          n86 = case shown="True" w265 {
            tunnel: [u8 5 u8 4] -> w264
            frame True {
            }
            frame False {
            }
          }
        }
        frame 5 {
          # "Waits for a reverse correlation that's close to the first correlation, but make sure it's in the right speed range."
          n87 = Unbundle By Name(w286) -> ("Detector Min Speed Count"=w285:i32)
          n88 = Unbundle By Name(w273) -> ("First Correlation"=w278:i32)
          n89 = Increment(x=w276) -> (x+1=w271:T14)
          n90 = Unbundle By Name(w271) -> ("First Detector Count"=w277:i32)
          n91 = Add(x=w281, y=w280) -> (x+y=w272:i32)
          n92 = Greater Or Equal?(x=w277, y=w285) -> (x >= y?=w284:bool)
          n93 = case shown="False" w284 {
            tunnel: [_ w302] -> w279
            tunnel: [u8 5 _] -> _
            tunnel: w283 -> [_ w301]
            tunnel: w282 -> [_ w298]
            tunnel: w278 -> [_ w289]
            tunnel: [_ w288] -> w274
            frame True {
            }
            frame False {
              n94 = Unbundle By Name(w298) -> ("Filter 1.Det 1"=w295:i32, "Filter 1.Det 1"=w297:i32, "Filter 1.Det 1"=w296:i32)
              n95 = To Fixed-Point(number=w289) -> (fixed-point=w291:fxp<+/-,32,32>)  [unwired: 1 in]
              n96 = Subtract(x=fxp<+,1,1> 1.0, y=w301) -> (x-y=w299:fxp<+,33,1>)
              n97 = Add(x=w297, y=w296) -> (x+y=w294:i32)
              n98 = Multiply(x=w299, y=w291) -> (x*y=w293:fxp<+/-,64,32>)
              n99 = Subtract(x=w295, y=w294) -> (x-y=w288:i32)
              n100 = To Fixed-Point(number=w288) -> (fixed-point=w290:fxp<+/-,32,32>)  [unwired: 1 in]
              n101 = Greater?(x=w290, y=w293) -> (0:w292:bool)
              n102 = case shown="True" w292 {
                tunnel: [u8 6 u8 5] -> w302
                frame True {
                }
                frame False {
                }
              }
            }
          }
          n103 = Bundle(cluster=w273, "Latest Correlation"=w274) -> (w275:T15)  [unwired: 1 in]
        }
        frame 6 {
          # "Waits for Boxcar 2 to reach the halfway point\nbetween Boxcars 1 and 3+4."
          n104 = Unbundle By Name(w314) -> ("Detector Min Speed Count"=w310:i32)
          n105 = Unbundle By Name(w330) -> ("Filter 1.Det 1"=w340:i32, "Filter 1.Det 1"=w343:i32, "Filter 1.Det 1"=w342:i32, "Filter 1.Det 1"=w334:i32)
          n106 = Unbundle By Name(w313) -> ("First Detector Count"=w311:i32)
          n107 = Increment(x=w313) -> (x+1=w324:T14)
          n108 = To Fixed-Point(number=w338) -> (fixed-point=w327:fxp<+/-,32,32>)  [unwired: 1 in]
          n109 = Decrement(x=w346) -> (x-1=w326:i32)
          n110 = Increment(x=w323) -> (x+1=w320:fxp<+,33,1>)
          n111 = Add(x=w343, y=w342) -> (x+y=w341:i32)
          n112 = Unbundle(w312) -> ("First Correlation"=w322:i32, "Latest Correlation"=w306:i32)
          n113 = To Fixed-Point(number=w322) -> (fixed-point=w321:fxp<+/-,32,32>)  [unwired: 1 in]
          n114 = Add(x=w340, y=w341) -> (x+y=w344:i32)
          n115 = Subtract(x=w340, y=w341) -> (x-y=w319:i32)
          n116 = To Fixed-Point(number=w334) -> (fixed-point=w329:fxp<+/-,32,32>)  [unwired: 1 in]
          n117 = Multiply(x=w321, y=w320) -> (x*y=w317:fxp<+/-,64,33>)
          n118 = To Fixed-Point(number=w337) -> (fixed-point=w328:fxp<+/-,32,32>)  [unwired: 1 in]
          n119 = To Fixed-Point(number=w344) -> (fixed-point=w331:fxp<+/-,32,32>)  [unwired: 1 in]
          n120 = Greater Or Equal?(x=w311, y=w310) -> (x >= y?=w309:bool)
          n121 = Multiply(x=w331, y=w327) -> (x*y=w339:fxp<+/-,64,64>)
          n122 = To Fixed-Point(number=w319) -> (fixed-point=w318:fxp<+/-,32,32>)  [unwired: 1 in]
          n123 = Scale By Power Of 2(n=i16 1, x=w328) -> (x*2^n=w335:fxp<+/-,32,32>)
          n124 = Max & Min(x=w319, y=w306) -> (max(x,y)=w305:i32)  [unwired: 1 out]
          n125 = Greater?(x=w318, y=w317) -> (0:w316:bool)
          n126 = Multiply(x=w329, y=w335) -> (x*y=w333:fxp<+/-,64,64>)
          n127 = Or(x=w316, y=w309) -> (x .or. y?=w315:bool)
          n128 = Less?(x=w339, y=w333) -> (x < y?=w325:bool)
          n129 = case shown="True" w325 {
            tunnel: [w351 u8 7 ("Det 3")] -> w345
            tunnel: w326 -> [w348 _]
            tunnel: w315 -> [w347 _]
            frame False {
              n130 = Less Or Equal To 0?(x=w348) -> (x <= 0?=w349:bool)
              n131 = Or(x=w347, y=w349) -> (x .or. y?=w350:bool)
              n132 = case shown="False" w350 {
                tunnel: [u8 6 ("Det 3") _] -> w351
                frame False {
                }
                frame True {
                  (unwired) u8 6 ("Det 3")
                }
              }
            }
            frame True {
            }
          }
          n133 = Bundle By Name(cluster=w312, "Latest Correlation"=w305) -> (w332:T15)
          n134 = Bundle By Name(cluster=w324, "Detector Gap Count"=0) -> (w308:T14)
        }
        frame 7 {
          # "q = ADC value / CSA sensitivity"
          # "Ensures the charge is good"
          n135 = Unbundle(w360) -> ("First Correlation"=w374:i32, "Latest Correlation"=w373:i32)
          n136 = Unbundle By Name(w375) -> ("High Charge Limit"=w354:fxp<+,32,-41>, "Low Charge Limit"=w371:fxp<+,32,-41>)
          n137 = Add(x=w374, y=w373) -> (x+y=w363:i32)
          n138 = Increment(x=w358) -> (x+1=w357:T14)
          n139 = Scale By Power Of 2(n=i16 -1, x=w363) -> (x*2^n=w361:i32)
          n140 = To Fixed-Point(number=w361) -> (fixed-point=w362:fxp<+/-,32,32>)  [unwired: 1 in]
          n141 = Multiply(x=w362, y=w372) -> (x*y=w366:fxp<+/-,47,32>)
          n142 = Multiply(x=w366, y=w365) -> (x*y=w356:fxp<+/-,64,-17>)
          n143 = Bundle(cluster=w360, "First Correlation"=w361) -> (w359:T15)  [unwired: 1 in]
          n144 = To Fixed-Point(fixed-point type=w354, number=w356) -> (fixed-point=w355:fxp<+,32,-41>)
          n145 = Less Or Equal?(x=w355, y=w354) -> (x <= y?=w370:bool)
          n146 = Greater Or Equal?(x=w355, y=w371) -> (x >= y?=w369:bool)
          n147 = And(x=w370, y=w369) -> (x .and. y?=w368:bool)
          n148 = case shown="True" w368 {
            tunnel: [u8 8 ("Det 3") _] -> w367
            frame True {
            }
            frame False {
              (unwired) u8 7 ("Det 3")
            }
          }
        }
        frame 8 {
          # "This section ensures that we only look for the particle\nwithin the speed bounds of the current filter"
          n149 = Increment(x=w379) -> (x+1=w378:T14)
          n150 = Unbundle By Name(w385) -> ("Gap Max Speed Count"=w383:i32)
          n151 = Unbundle By Name(w378) -> ("Detector Gap Count"=w384:i32)
          n152 = Greater Or Equal?(x=w384, y=w383) -> (x >= y?=w382:bool)
          n153 = case shown="True" w382 {
            tunnel: [u8 9 u8 8] -> w381
            frame True {
            }
            frame False {
            }
          }
        }
        frame 9 {
          # "Waits for a second detector correlation that's close to the\nfirst correlation, but make sure it's in the right speed range."
          n154 = Unbundle By Name(w391) -> ("First Correlation"=w394:i32)
          n155 = Increment(x=w392) -> (x+1=w389:T14)
          n156 = Unbundle By Name(w402) -> ("Gap Min Speed Count"=w401:i32)
          n157 = Unbundle By Name(w389) -> ("Detector Gap Count"=w393:i32)
          n158 = Add(x=w397, y=w396) -> (x+y=w390:i32)
          n159 = Greater Or Equal?(x=w393, y=w401) -> (x >= y?=w400:bool)
          n160 = case shown="False" w400 {
            tunnel: [_ w417] -> w395
            tunnel: w399 -> [_ w416]
            tunnel: w398 -> [_ w413]
            tunnel: w394 -> [_ w404]
            frame True {
              (unwired) u8 9
            }
            frame False {
              n161 = Unbundle By Name(w413) -> ("Filter 1.Det 1"=w410:i32, "Filter 1.Det 1"=w412:i32, "Filter 1.Det 1"=w411:i32)
              n162 = To Fixed-Point(number=w404) -> (fixed-point=w406:fxp<+/-,32,32>)  [unwired: 1 in]
              n163 = Subtract(x=fxp<+,1,1> 1.0, y=w416) -> (x-y=w414:fxp<+,33,1>)
              n164 = Add(x=w412, y=w411) -> (x+y=w409:i32)
              n165 = Multiply(x=w414, y=w406) -> (x*y=w408:fxp<+/-,64,32>)
              n166 = Subtract(x=w409, y=w410) -> (x-y=w403:i32)
              n167 = To Fixed-Point(number=w403) -> (fixed-point=w405:fxp<+/-,32,32>)  [unwired: 1 in]
              n168 = Greater?(x=w405, y=w408) -> (0:w407:bool)
              n169 = case shown="True" w407 {
                tunnel: [u8 10 u8 9] -> w417
                frame True {
                }
                frame False {
                }
              }
            }
          }
        }
        frame 10 {
          # "Waits for Boxcar 2 to reach the halfway point\nbetween Boxcars 1 and 3+4."
          n170 = Unbundle By Name(w444) -> ("Filter 1.Det 2"=w453:i32, "Filter 1.Det 2"=w456:i32, "Filter 1.Det 2"=w455:i32, "Filter 1.Det 2"=w447:i32)
          n171 = Increment(x=w428) -> (x+1=w423:T14)
          n172 = To Fixed-Point(number=w451) -> (fixed-point=w441:fxp<+/-,32,32>)  [unwired: 1 in]
          n173 = Unbundle By Name(w427) -> ("Gap Min Speed Count"=w425:i32)
          n174 = Unbundle By Name(w428) -> ("Detector Gap Count"=w426:i32)
          n175 = Decrement(x=w459) -> (x-1=w440:i32)
          n176 = Increment(x=w438) -> (x+1=w434:fxp<+,33,1>)
          n177 = Add(x=w456, y=w455) -> (x+y=w454:i32)
          n178 = Unbundle(w437) -> ("First Correlation"=w436:i32)  [unwired: 1 out]
          n179 = To Fixed-Point(number=w436) -> (fixed-point=w435:fxp<+/-,32,32>)  [unwired: 1 in]
          n180 = Add(x=w453, y=w454) -> (x+y=w457:i32)
          n181 = Subtract(x=w454, y=w453) -> (x-y=w433:i32)
          n182 = To Fixed-Point(number=w447) -> (fixed-point=w443:fxp<+/-,32,32>)  [unwired: 1 in]
          n183 = Multiply(x=w435, y=w434) -> (x*y=w431:fxp<+/-,64,33>)
          n184 = To Fixed-Point(number=w450) -> (fixed-point=w442:fxp<+/-,32,32>)  [unwired: 1 in]
          n185 = To Fixed-Point(number=w457) -> (fixed-point=w445:fxp<+/-,32,32>)  [unwired: 1 in]
          n186 = Multiply(x=w445, y=w441) -> (x*y=w452:fxp<+/-,64,64>)
          n187 = To Fixed-Point(number=w433) -> (fixed-point=w432:fxp<+/-,32,32>)  [unwired: 1 in]
          n188 = Scale By Power Of 2(n=i16 1, x=w442) -> (x*2^n=w448:fxp<+/-,32,32>)
          n189 = Greater Or Equal?(x=w426, y=w425) -> (x >= y?=w424:bool)
          n190 = Greater?(x=w432, y=w431) -> (0:w430:bool)
          n191 = Multiply(x=w443, y=w448) -> (x*y=w446:fxp<+/-,64,64>)
          n192 = Or(x=w430, y=w424) -> (x .or. y?=w429:bool)
          n193 = Greater?(x=w452, y=w446) -> (0:w439:bool)
          n194 = case shown="True" w439 {
            tunnel: [w464 u8 11 ("Det 3")] -> w458
            tunnel: w440 -> [w461 _]
            tunnel: w429 -> [w460 _]
            frame False {
              n195 = Less Or Equal To 0?(x=w461) -> (x <= 0?=w462:bool)
              n196 = Or(x=w460, y=w462) -> (x .or. y?=w463:bool)
              n197 = case shown="False" w463 {
                tunnel: [u8 10 ("Det 3") _] -> w464
                frame False {
                }
                frame True {
                  (unwired) u8 10 ("Det 3")
                }
              }
            }
            frame True {
            }
          }
          n198 = Bundle By Name(cluster=w423, "Second Detector Count"=0) -> (w422:T14)
        }
        frame 11 {
          # "This section ensures that we only look for the particle\nwithin the speed bounds of the current filter"
          n199 = Increment(x=w469) -> (x+1=w468:T14)
          n200 = Unbundle By Name(w475) -> ("Detector Max Speed Count"=w473:i32)
          n201 = Unbundle By Name(w468) -> ("Second Detector Count"=w474:i32)
          n202 = Greater Or Equal?(x=w474, y=w473) -> (x >= y?=w472:bool)
          n203 = case shown="True" w472 {
            tunnel: [u8 12 u8 11] -> w471
            frame True {
            }
            frame False {
            }
          }
        }
        frame 12 {
          # "Waits for a reverse correlation that's close to the first correlation, but make sure it's in the right speed range."
          n204 = Unbundle By Name(w492) -> ("Detector Min Speed Count"=w491:i32)
          n205 = Unbundle By Name(w478) -> ("First Correlation"=w484:i32)
          n206 = Increment(x=w482) -> (x+1=w480:T14)
          n207 = Unbundle By Name(w480) -> ("Second Detector Count"=w483:i32)
          n208 = Add(x=w487, y=w486) -> (x+y=w481:i32)
          n209 = Greater Or Equal?(x=w483, y=w491) -> (x >= y?=w490:bool)
          n210 = case shown="False" w490 {
            tunnel: [_ w507] -> w485
            tunnel: w489 -> [_ w506]
            tunnel: w488 -> [_ w503]
            tunnel: w484 -> [_ w494]
            frame True {
              (unwired) u8 12
            }
            frame False {
              n211 = Unbundle By Name(w503) -> ("Filter 1.Det 2"=w500:i32, "Filter 1.Det 2"=w502:i32, "Filter 1.Det 2"=w501:i32)
              n212 = To Fixed-Point(number=w494) -> (fixed-point=w496:fxp<+/-,32,32>)  [unwired: 1 in]
              n213 = Subtract(x=fxp<+,1,1> 1.0, y=w506) -> (x-y=w504:fxp<+,33,1>)
              n214 = Add(x=w502, y=w501) -> (x+y=w499:i32)
              n215 = Multiply(x=w504, y=w496) -> (x*y=w498:fxp<+/-,64,32>)
              n216 = Subtract(x=w500, y=w499) -> (x-y=w493:i32)
              n217 = To Fixed-Point(number=w493) -> (fixed-point=w495:fxp<+/-,32,32>)  [unwired: 1 in]
              n218 = Greater?(x=w495, y=w498) -> (0:w497:bool)
              n219 = case shown="True" w497 {
                tunnel: [u8 13 u8 12] -> w507
                frame True {
                }
                frame False {
                }
              }
            }
          }
        }
        frame 13 {
          # "Waits for Boxcar 2 to reach the halfway point\nbetween Boxcars 1 and 3+4."
          n220 = Unbundle By Name(w517) -> ("Detector Min Speed Count"=w514:i32)
          n221 = Unbundle By Name(w532) -> ("Filter 1.Det 2"=w541:i32, "Filter 1.Det 2"=w544:i32, "Filter 1.Det 2"=w543:i32, "Filter 1.Det 2"=w535:i32)
          n222 = Unbundle By Name(w516) -> ("Second Detector Count"=w515:i32)
          n223 = Increment(x=w516) -> (x+1=w526:T14)
          n224 = To Fixed-Point(number=w539) -> (fixed-point=w529:fxp<+/-,32,32>)  [unwired: 1 in]
          n225 = Decrement(x=w547) -> (x-1=w528:i32)
          n226 = Increment(x=w525) -> (x+1=w522:fxp<+,33,1>)
          n227 = Add(x=w544, y=w543) -> (x+y=w542:i32)
          n228 = Unbundle(w510) -> ("First Correlation"=w524:i32)  [unwired: 1 out]
          n229 = To Fixed-Point(number=w524) -> (fixed-point=w523:fxp<+/-,32,32>)  [unwired: 1 in]
          n230 = Add(x=w541, y=w542) -> (x+y=w545:i32)
          n231 = Subtract(x=w541, y=w542) -> (x-y=w521:i32)
          n232 = To Fixed-Point(number=w535) -> (fixed-point=w531:fxp<+/-,32,32>)  [unwired: 1 in]
          n233 = Multiply(x=w523, y=w522) -> (x*y=w519:fxp<+/-,64,33>)
          n234 = To Fixed-Point(number=w538) -> (fixed-point=w530:fxp<+/-,32,32>)  [unwired: 1 in]
          n235 = To Fixed-Point(number=w545) -> (fixed-point=w533:fxp<+/-,32,32>)  [unwired: 1 in]
          n236 = Greater Or Equal?(x=w515, y=w514) -> (x >= y?=w512:bool)
          n237 = Multiply(x=w533, y=w529) -> (x*y=w540:fxp<+/-,64,64>)
          n238 = To Fixed-Point(number=w521) -> (fixed-point=w520:fxp<+/-,32,32>)  [unwired: 1 in]
          n239 = Scale By Power Of 2(n=i16 1, x=w530) -> (x*2^n=w536:fxp<+/-,32,32>)
          n240 = Greater?(x=w520, y=w519) -> (0:w518:bool)
          n241 = Multiply(x=w531, y=w536) -> (x*y=w534:fxp<+/-,64,64>)
          n242 = Or(x=w518, y=w512) -> (x .or. y?=w513:bool)
          n243 = Less?(x=w540, y=w534) -> (x < y?=w527:bool)
          n244 = case shown="True" w527 {
            tunnel: [w552 u8 14 ("Det 3")] -> w546
            tunnel: w528 -> [w549 _]
            tunnel: w513 -> [w548 _]
            frame False {
              n245 = Less Or Equal To 0?(x=w549) -> (x <= 0?=w550:bool)
              n246 = Or(x=w548, y=w550) -> (x .or. y?=w551:bool)
              n247 = case shown="False" w551 {
                tunnel: [u8 13 ("Det 3") _] -> w552
                frame False {
                }
                frame True {
                  (unwired) u8 13 ("Det 3")
                }
              }
            }
            frame True {
            }
          }
        }
        frame 14 {
          # "Look carefully at the way the Armed variable is treated in here.\nIf One Shot implies Armed (ie, it's okay to let a particle through),\nthe particle is allowed to go through, but Armed is turned off."
          # "v = clockspeed * distance / speed count"
          # "1/2mv^2 = Vq\ntherefore\nm = 2Vq/v^2"
          n248 = Unbundle By Name(w556) -> ("First Detector Count"=w555:i32)
          n249 = Unbundle By Name(w584) -> ("High Velocity Limit"=w571:fxp<+,18,18>, "Low Velocity Limit"=w572:fxp<+,18,18>, "High Mass Limit"=w580:fxp<+,32,-37>, "Low Mass Limit"=w560:fxp<+,32,-37>, "High Voltage"=w575:fxp<+,32,22>)
          n250 = Multiply(x=w575, y=w562) -> (x*y=w581:fxp<+,64,-19>)
          n251 = To Fixed-Point(number=w555) -> (fixed-point=w570:fxp<+/-,32,32>)  [unwired: 1 in]
          n252 = To Fixed-Point(number=w555) -> (fixed-point=w563:fxp<+/-,32,32>)  [unwired: 1 in]
          n253 = Square(x=w563) -> (x^2=w564:fxp<+,63,63>)
          n254 = Multiply(x=w571, y=w570) -> (x*y=w569:fxp<+/-,50,50>)
          n255 = Multiply(x=w570, y=w572) -> (x*y=w568:fxp<+/-,50,50>)
          n256 = Multiply(x=w583, y=w564) -> (x*y=w582:fxp<+,64,19>)
          n257 = To Fixed-Point(fixed-point type=fxp<+,32,-13> 0.0, number=w582) -> (fixed-point=w558:fxp<+,32,-13>)
          n258 = Greater Or Equal?(x=w569, y=w561) -> (x >= y?=w579:bool)
          n259 = Less Or Equal?(x=w568, y=w561) -> (x <= y?=w578:bool)
          n260 = Multiply(x=w581, y=w558) -> (x*y=w565:fxp<+,64,-32>)
          n261 = Scale By Power Of 2(n=i16 1, x=w565) -> (x*2^n=w559:fxp<+,64,-32>)
          n262 = Less Or Equal?(x=w559, y=w580) -> (x <= y?=w577:bool)
          n263 = Greater Or Equal?(x=w559, y=w560) -> (x >= y?=w576:bool)
          n264 = Compound Arithmetic op=AND(w579, w578, w577, w576, w567) -> (w566:bool)
          n265 = case shown="True" w566 {
            tunnel: [u8 15 ("Det 3") _] -> w573
            frame True {
            }
            frame False {
              (unwired) u8 14 ("Det 3")
            }
          }
        }
        frame 15 {
          # "To keep the names in the distance cluster from\ncorrupting the names of the speed counts cluster.\nThis really shouldn't happen, but it does."
          n266 = Unbundle By Name(w594) -> ("First Detector Count"=w600:i32)
          n267 = To Fixed-Point(number=w600) -> (fixed-point=w610:fxp<+/-,32,32>)  [unwired: 1 in]
          n268 = Multiply(x=w610, y=w609) -> (x*y=w608:T19)
          n269 = To Long Integer(number=w608) -> (32bit integer=w607:T20)
          n270 = Scale By Power Of 2(n=i16 -1, x=w598) -> (x*2^n=w599:i32)
          n271 = Subtract(x=w607, y=w606) -> (x-y=w605:T20)
          n272 = Subtract(x=w605, y=w599) -> (x-y=w596:T20)
          n273 = Unbundle By Name(w596) -> ("Distance to DCS 1"=w602:i32)
          n274 = Unbundle By Name(w596) -> ("Distance to PSU"=w593:i32, "Distance to end of PSU"=w592:i32, "Distance to DCS 2"=w591:i32, "Distance to front of LEIL Chamber"=w587:i32)
          n275 = Add(x=w602, y=w603) -> (x+y=w601:i32)
          n276 = To Long Integer(number=w587) -> (32bit integer=w586:i32)
          n277 = To Long Integer(number=w593) -> (32bit integer=w590:i32)
          n278 = To Long Integer(number=w592) -> (32bit integer=w589:i32)
          n279 = To Long Integer(number=w591) -> (32bit integer=w588:i32)
          n280 = Bundle(cluster=w594, "First Detector Count"=w590, "Detector Gap Count"=w589, "Second Detector Count"=w588, "Second Detector Final Count"=w586) -> (w595:T14)
        }
        frame 16 {
          n281 = Decrement(x=w631) -> (x-1=w630:T14)
          n282 = Unbundle(w630) -> ("First Detector Count"=w625:i32, "Detector Gap Count"=w623:i32, "Second Detector Count"=w620:i32, "Second Detector Final Count"=w618:i32)
          n283 = Add(x=w620, y=w629) -> (x+y=w621:i32)
          n284 = Add(x=w618, y=w629) -> (x+y=w617:i32)
          n285 = Less Or Equal To 0?(x=w620) -> (x <= 0?=w619:bool)
          n286 = Greater Or Equal To 0?(x=w617) -> (x >= 0?=w615:bool)
          n287 = Less Or Equal To 0?(x=w625) -> (x <= 0?=w624:bool)
          n288 = Less Or Equal To 0?(x=w618) -> (x <= 0?=w616:bool)
          n289 = Greater Or Equal To 0?(x=w621) -> (x >= 0?=w612:bool)
          n290 = Greater Or Equal To 0?(x=w623) -> (x >= 0?=w622:bool)
          n291 = And(x=w616, y=w615) -> (x .and. y?=w626:bool)
          n292 = And(x=w624, y=w622) -> (x .and. y?=w628:bool)
          n293 = And(x=w619, y=w612) -> (x .and. y?=w627:bool)
          n294 = And(x=w611, y=w615) -> (x .and. y?=w613:bool)
          n295 = Or(x=w613, y=w612) -> (x .or. y?=w614:bool)
          n296 = case shown="False" w614 {
            tunnel: [u8 16 ("Det 3") _] -> w632
            frame True {
            }
            frame False {
            }
          }
        }
      }
      n297 = disable-structure shown="Disabled" {
        disable-tunnel: w158 -> [w644 w656]
        disable-tunnel: [w640 w655] -> w154
        disable-tunnel: [w642 _] -> w153
        disable-tunnel: w152 -> [w643 _]
        frame Disabled {
          n298 = case shown="1, Default" w644 {
            selector: w644 -> [_ w650]
            tunnel: [w647 w648] -> w641
            tunnel: w643 -> [w647 w649]
            frame 0 {
            }
            frame 1, Default {
              n299 = case shown="1, Default" w649 {
                selector: w649 -> [_ w653]
                tunnel: w650 -> [w651 w654]
                tunnel: [w651 w652] -> w648
                frame 0 {
                }
                frame 1, Default {
                  n300 = Max & Min(x=w654, y=w653) -> (min(x,y)=w652:i32)  [unwired: 1 out]
                }
              }
            }
          }
          n301 = Less Than 0?(x=w641) -> (x < 0?=w640:bool)
          n302 = case shown="False" w640 {
            tunnel: w641 -> [w646 _]
            tunnel: [w645 _] -> w642
            frame False {
              n303 = Decrement(x=w646) -> (x-1=w645:i32)
            }
            frame True {
            }
          }
        }
        frame Enabled {
          n304 = Not Equal To 0?(x=w656) -> (x != 0?=w655:bool)
        }
      }
      n305 = case shown="False" w154 {
        tunnel: w157 -> [_ w639]
        tunnel: [w634 w639] -> w156
        tunnel: w155 -> [w635 _]
        frame False {
          n306 = case shown="1, Default" w635 {
            selector: w635 -> [w636 w638]
            tunnel: [w636 w637] -> w634
            frame 0 {
            }
            frame 1, Default {
              n307 = Decrement(x=w638) -> (x-1=w637:u16)
            }
          }
        }
        frame True {
        }
      }
    }
    n308 = Delete From Array(array=w66) -> (array with subset deleted=w65:cluster{"Det 1":i16, "Det 2":i16}[])  [unwired: 2 in, 1 out]
    n309 = case shown="True" "Calibrate" {
      tunnel: w75 -> [w137 _]
      tunnel: [w137 w138] -> w113
      tunnel: w61 -> [_ w138]
      frame False {
      }
      frame True {
      }
    }
    n310 = Or Array Elements(Boolean array=w85) -> (logical OR=w79:bool)
    n311 = Greater Than 0?(x=w107) -> (x > 0?=w98:bool[])
    n312 = Not(x=w79) -> (.not. x?=w84:bool)
    n313 = Or Array Elements(Boolean array=w98) -> (logical OR=w53:bool)
    n314 = Or Array Elements(Boolean array=w88) -> (logical OR=w60:bool)
    n315 = Or Array Elements(Boolean array=w87) -> (logical OR=w57:bool)
    n316 = Or Array Elements(Boolean array=w86) -> (logical OR=w55:bool)
    n317 = And(x=w84, y=w82) -> (x .and. y?=w83:bool)
    n318 = local write "Armed"(w83) -> ()
    n319 = xnode ("Handshake Write")("Data"=w55, "Input Valid"=TRUE) -> ()  [unwired: 1 in, 2 out]
    n320 = xnode ("Handshake Write")("Data"=w60, "Input Valid"=TRUE) -> ()  [unwired: 1 in, 2 out]
    n321 = xnode ("Handshake Write")("Data"=w57, "Input Valid"=TRUE) -> ()  [unwired: 1 in, 2 out]
    n322 = xnode ("Handshake Write")("Data"=w53, "Input Valid"=TRUE) -> ()  [unwired: 1 in, 2 out]
  }
  n323 = timed-loop {
    timing: w32 -> [_]
    timing-out: [_] -> w31
    shift-right: [w672] -> _
    shift-left: w27 -> [w681]
    shift-right: [w674] -> _
    shift-left: w25 -> [w679]
    stop <- _ stop-if-true
    w659 = TRUE ("IO Module\\PFI Enable")
    n324 = xnode "FPGA I/O Node"() -> ("IO Module\\AI 0"=w678:i16, "IO Module\\AI 1"=w677:i16)  [unwired: 2 in, 2 out]
    n325 = xnode ("Handshake Read")("Ready for Output"=TRUE) -> ("Data"=w667:bool)  [unwired: 1 in, 2 out]
    n326 = xnode ("Handshake Read")("Ready for Output"=TRUE) -> ("Data"=w663:bool)  [unwired: 1 in, 2 out]
    n327 = Bundle("IO Module\\AI 0"=w678, "IO Module\\AI 1"=w677) -> (w676:T21)  [unwired: 1 in]
    n328 = xnode ("Handshake Read")("Ready for Output"=TRUE) -> ("Data"=w666:bool)  [unwired: 1 in, 2 out]
    n329 = Add(x=w676, y=w681) -> (x+y=w680:T7)
    n330 = Insert Into Array(array=w679, index=0, new element=w676) -> (w675:cluster{"Det 1":i16, "Det 2":i16}[])
    n331 = xnode ("Handshake Read")("Ready for Output"=TRUE) -> ("Data"=w660:bool)  [unwired: 1 in, 2 out]
    n332 = Delete From Array(array=w675) -> (deleted portion=w673:cluster{"Det 1":i16, "Det 2":i16}, array with subset deleted=w674:cluster{"Det 1":i16, "Det 2":i16}[])  [unwired: 2 in]
    n333 = Subtract(x=w680, y=w673) -> (x-y=w672:T7)
    n334 = Unbundle(w672) -> ("Det 1"=w670:i32, "Det 2"=w668:i32)
    n335 = xnode "FPGA I/O Node"("IO Module\\PFI 0 WE"=w659, "IO Module\\PFI 1 WE"=w659, "IO Module\\PFI 2 WE"=w659, "IO Module\\PFI 3 WE"=w659) -> ()  [unwired: 4 in, 4 out]
    n336 = xnode "FPGA I/O Node"("IO Module\\PFI 0 Wr Data"=w660, "IO Module\\PFI 1 Wr Data"=w663, "IO Module\\PFI 2 Wr Data"=w666, "IO Module\\PFI 3 Wr Data"=w667) -> ()  [unwired: 4 in, 4 out]
    n337 = xnode ("Handshake Write")("Data"=w670, "Input Valid"=TRUE) -> ()  [unwired: 1 in, 2 out]
    n338 = xnode ("Handshake Write")("Data"=w668, "Input Valid"=TRUE) -> ()  [unwired: 1 in, 2 out]
  }
  n339 = node-c288(w31) -> ()
  n340 = node-c288(w38) -> ()
